vi "D_point2line.vi"(5 "slope":dbl, 7 "intercept":dbl, 10 "X Array":ext[](array[numeric]), 11 "Y Array":ext[](array[numeric])) -> (0 "Y_online":ext[](array[numeric]), 1 "X_online":ext[](array[numeric]), 3 "D":ext[](array[numeric]))   [LabVIEW 2017]
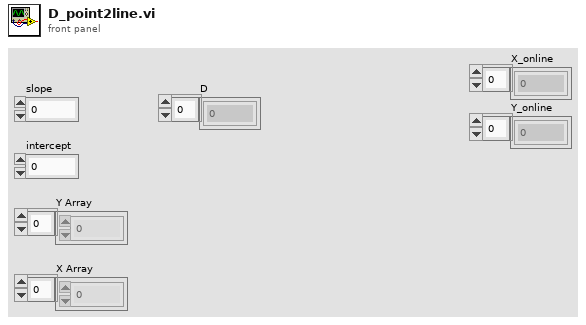
[diagram p1: front panel]
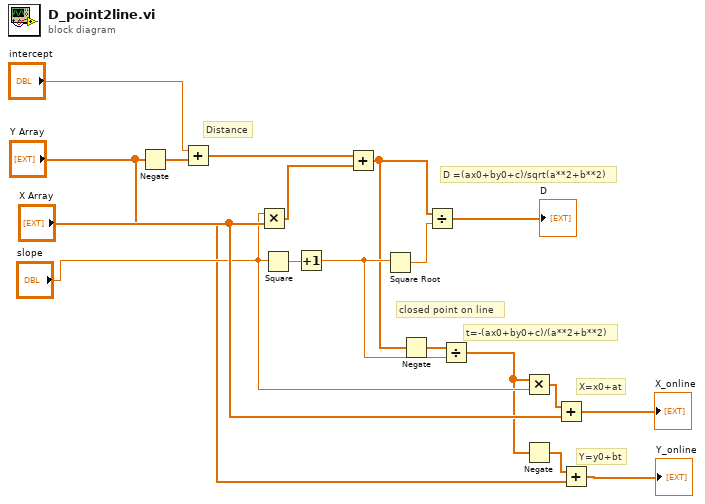
[diagram p0: block diagram]
diagram:
  # "D =(ax0+by0+c)/sqrt(a**2+b**2)"
  # "Y=y0+bt"
  # "X=x0+at"
  # "t=-(ax0+by0+c)/(a**2+b**2)"
  # "closed point on line"
  # "Distance"
  n1 = Negate(x="Y Array") -> (-x=w15:ext[])
  n2 = Add(x="intercept", y=w15) -> (x+y=w16:ext[])
  n3 = Multiply(x="slope", y="X Array") -> (x*y=w17:ext[])
  n4 = Square(x="slope") -> (x^2=w13:dbl)
  n5 = Increment(x=w13) -> (x+1=w12:dbl)
  n6 = Add(x=w16, y=w17) -> (x+y=w11:ext[])
  n7 = Square Root(x=w12) -> (sqrt(x)=w18:dbl)
  n8 = Negate(x=w11) -> (-x=w10:ext[])
  n9 = Divide(x=w11, y=w18) -> (x/y=→"D":ext[])
  n10 = Divide(x=w10, y=w12) -> (x/y=w6:ext[])
  n11 = Multiply(x=w6, y="slope") -> (x*y=w8:ext[])
  n12 = Negate(x=w6) -> (-x=w5:ext[])
  n13 = Add(x=w8, y="X Array") -> (x+y=→"X_online":ext[])
  n14 = Add(x=w5, y="Y Array") -> (x+y=→"Y_online":ext[])
